vi "Check VC++ Redist.vi"(8 "Error In":errorcluster) -> (0 "Error Out":errorcluster, 2 "Installed?":bool)   [LabVIEW 2011, in "LVH-Adept.lvlib"]
uses:
  <vilib>/LabVIEW Hacker/Adept/LVH-Adept.lvlib
  <vilib>/registry/registry.llb/Registry SAM.ctl
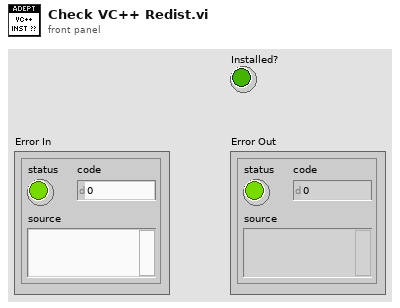
[diagram p1: front panel]
types:
  T1 = typedef "Registry SAM.ctl" = enum32{"KEY_QUERY_VALUE", "KEY_SET_VALUE", "KEY_CREATE_SUB_KEY", "KEY_ENUMERATE_SUB_KEYS", "KEY_NOTIFY", "KEY_CREATE_LINK", "KEY_READ", "KEY_WRITE", "KEY_ALL_ACCESS", "KEY_READ | KEY_WRITE"}
  T2 = typedef "Registry refnum.ctl" = refnum<k1>
  T3 = cluster{"numSubKeys":i32, "maxSubKeyLen":i32, "maxSubKeyClassLen":i32}
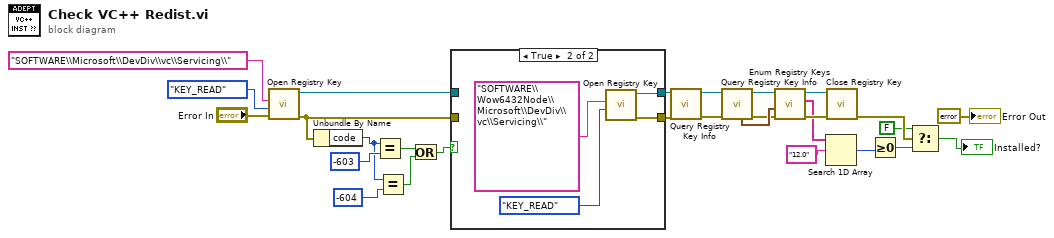
[diagram p0: block diagram]
diagram:
  n1 = call <vilib>:"Open Registry Key.vi"("error in (no error)"="Error In", "security access mask (KEY_READ | KEY_WRITE)"=Registry_SAM."KEY_READ", "subkey"="SOFTWARE\\Microsoft\\DevDiv\\vc\\Servicing\\") -> ("error out"=w25:errorcluster, "refnum out"=w23:T2)  [unwired: 7 in]
  n2 = Unbundle By Name(w25) -> ("code"=w18:i32)
  n3 = Equal?(x=w18, y=-603) -> (x = y?=w20:bool)
  n4 = Equal?(x=w18, y=-604) -> (x = y?=w17:bool)
  n5 = Or(x=w20, y=w17) -> (x .or. y?=w21:bool)
  n6 = case shown="True" w21 {
    tunnel: w25 -> [w29 _]
    tunnel: [w30 w33] -> w24
    tunnel: w23 -> [w30 _]
    tunnel: [w29 w32] -> w22
    frame False {
      # "Found x32 Entry"
    }
    frame True {
      n7 = call <vilib>:"Open Registry Key.vi"("security access mask (KEY_READ | KEY_WRITE)"=Registry_SAM."KEY_READ", "subkey"="SOFTWARE\\Wow6432Node\\Microsoft\\DevDiv\\vc\\Servicing\\") -> ("error out"=w32:errorcluster, "refnum out"=w33:T2)  [unwired: 8 in]
    }
  }
  n8 = call <vilib>:"Query Registry Key Info.vi"("error in (no error)"=w22, "refnum"=w24) -> ("error out"=w13:errorcluster, "refnum out"=w14:T2)  [unwired: 5 in, 3 out]
  n9 = call <vilib>:"Query Registry Key Info.vi"("error in (no error)"=w13, "refnum"=w14) -> ("error out"=w11:errorcluster, "refnum out"=w15:T2, "subkey info"=w12:T3)  [unwired: 5 in, 2 out]
  n10 = call <vilib>:"Enum Registry Keys.vi"("error in (no error)"=w11, "subkey info"=w12, "refnum"=w15) -> ("error out"=w9:errorcluster, "subkeys"=w8:string[], "refnum out"=w10:T2)  [unwired: 6 in]
  n11 = Search 1D Array(1D array=w8, element="12.0") -> (index of element=w6:i32)  [unwired: 1 in]
  n12 = call <vilib>:"Close Registry Key.vi"("error in (no error)"=w9, "refnum"=w10) -> ("error out"=w5:errorcluster)  [unwired: 5 in]
  n13 = Greater Or Equal To 0?(x=w6) -> (x >= 0?=w4:bool)
  n14 = Select(t=FALSE, s=w5, f=w4) -> (s? t:f=→"Installed?":bool)
  "Error Out" <- errorcluster {"status"=FALSE, "code"=0, "source"=""} ("Error Out")
